vi "Merge_into_Array_cluster.vi"(1 "Index":i32, 2 "1D Array Insert":cluster{"X":sgl, "Y":sgl}[](array[cluster]), 3 "1D Array":cluster{"X":sgl, "Y":sgl}[](array[cluster]), 4 "2D Array":cluster{"X":sgl, "Y":sgl}[][](array[cluster])) -> (0 "Output Array":cluster{"X":sgl, "Y":sgl}[][](array[cluster]))   [LabVIEW 2015]
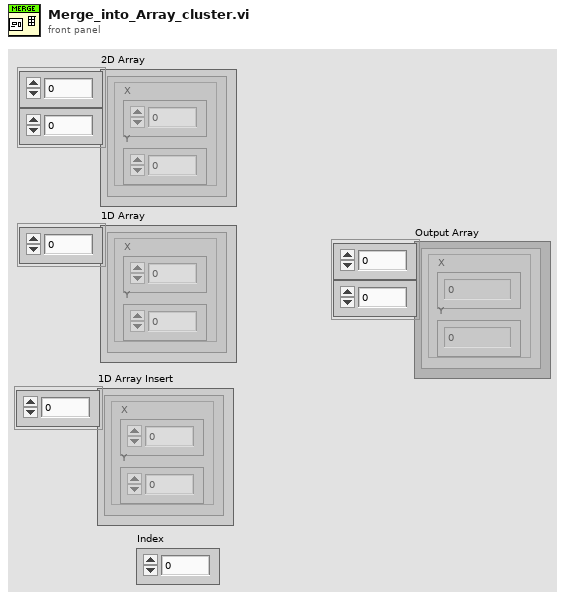
[diagram p1: front panel]
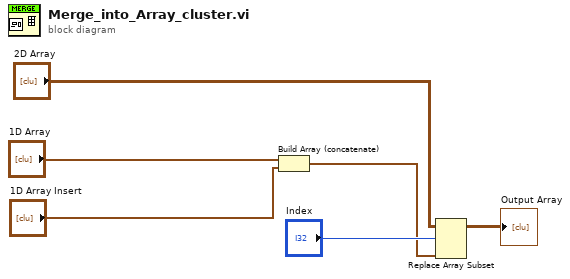
[diagram p0: block diagram]
diagram:
  n1 = Build Array (concatenate)("1D Array", "1D Array Insert") -> (w3:cluster{"X":sgl, "Y":sgl}[])
  n2 = Replace Array Subset(array="2D Array", new element=w3, index (row)="Index") -> (→"Output Array":cluster{"X":sgl, "Y":sgl}[][])  [unwired: 1 in]
